vi "CleanupReferences.vi"(5 "ActorRef":refnum<vi>, 7 "ActorLightIn":refnum<class "YActor.lvclass">, 10 "ArrayIn":variant[](array[variant]), 11 "CmdQ":refnum<queue>) -> ()   [LabVIEW 2021, in "YActor.lvclass"]
uses:
  YActor.lvclass
  CmdCtrl.ctl
  AsyncErrorHandling.ctl
  CallMode.ctl
  InlineReferencePool.ctl
  ActorPoolFunctions.ctl
  YActor.lvclass/YActor.ctl
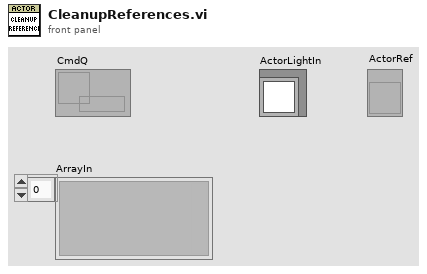
[diagram p1: front panel]
types:
  T1 = typedef "YActor.lvclass/ActorPoolFunctions.ctl" = enum16{"Add", "GetAll", "Delete"}
  T2 = typedef "YActor.lvclass/InlineReferencePool.ctl" = enum16{"Add", "ClearAll?"}
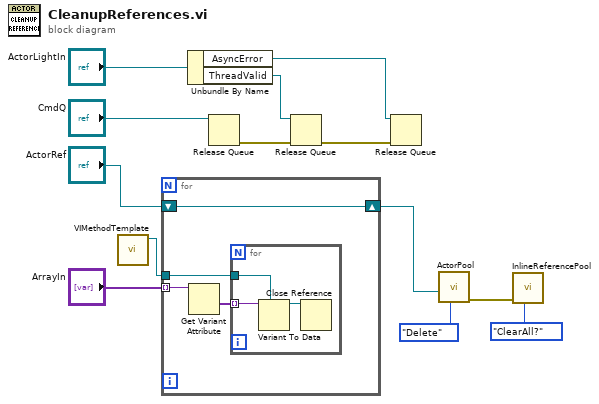
[diagram p0: block diagram]
diagram:
  n1 = call "VIMethodTemplate.vi"() -> ("VI out"=w10:refnum<vi>)  [unwired: 11 in]
  n2 = for {
    tunnel: "ArrayIn" -> [w17] mode=indexing
    tunnel: w10 -> [w15]
    shift-right: [w14] -> w2
    shift-left: "ActorRef" -> [w14]
    n3 = Get Variant Attribute(Variant=w17) -> (values=w16:variant[])  [unwired: 3 in, 3 out]
    n4 = for {
      tunnel: w16 -> [w20] mode=indexing
      tunnel: w15 -> [w19]
      n5 = Variant To Data(type=w19, Variant=w20) -> (data=w18:refnum<vi>)  [unwired: 1 in, 1 out]
      n6 = Close Reference(reference=w18) -> ()  [unwired: 1 in, 1 out]
    }
  }
  n7 = Unbundle By Name("ActorLightIn") -> ("AsyncError"=w7:refnum<queue>, "ThreadValid"=w6:refnum<queue>)
  n8 = Release Queue(queue="CmdQ") -> (error out=w13:errorcluster)  [unwired: 2 in, 2 out]
  n9 = Release Queue(queue=w6, error in (no error)=w13) -> (error out=w12:errorcluster)  [unwired: 1 in, 2 out]
  n10 = Release Queue(queue=w7, error in (no error)=w12) -> ()  [unwired: 1 in, 3 out]
  n11 = call "ActorPool.vi"("Functions"=ActorPoolFunctions."Delete", "ActorRef"=w2) -> ("ErrorOut"=w11:errorcluster)  [unwired: 7 in, 2 out]
  n12 = call "InlineReferencePool.vi"("functions"=InlineReferencePool."ClearAll?", "error in (no error)"=w11) -> ()  [unwired: 8 in, 2 out]
